vi "Icon Merge Layers.vi"(8 "error in (no error)":errorcluster, 11 "VI Refnum in":refnum<vi>) -> (0 "error out":errorcluster, 3 "VI Refnum out":refnum<vi>)   [LabVIEW 2019, in "Builtins.lvlib"]
doc: "Merges all VI icon layers to avoid icon template collisions.\n\nCreated by: Ryan Pacini"
uses:
  Builtins.lvlib
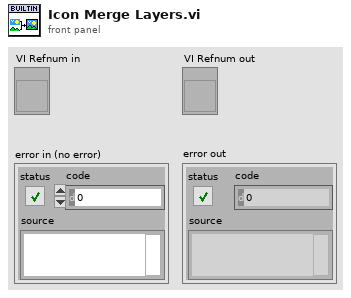
[diagram p1: front panel]
types:
  T1 = typedef "imagedata.ctl" = cluster{"image type":i32, "image depth":i32, "image":u8[], "mask":u8[], "colors":u32[], "Rectangle":cluster{"left":i16, "top":i16, "right":i16, "bottom":i16}}
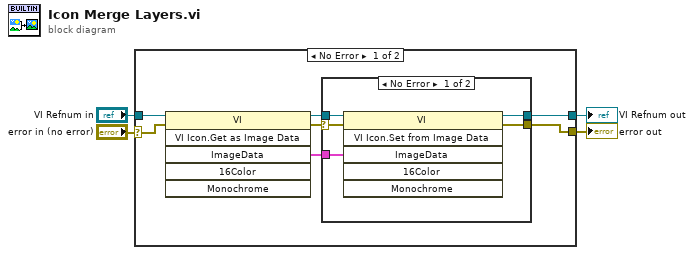
[diagram p0: block diagram]
diagram:
  n1 = case shown="No Error" "error in (no error)" {
    selector: "error in (no error)" -> [w11 w19]
    tunnel: "VI Refnum in" -> [w10 w20]
    tunnel: [w9 w20] -> w2
    tunnel: [w5 w19] -> w1
    frame No Error {
      n2 = invoke class="VI" method="VI Icon.Get as Image Data"(reference=w10, error in=w11) -> (reference out=w6:refnum<vi>, error out=w8:errorcluster, "ImageData"=w7:T1)  [unwired: 4 in, 3 out]
      n3 = case shown="No Error" w8 {
        selector: w8 -> [w14 w18]
        tunnel: w6 -> [w16 w17]
        tunnel: w7 -> [w15 _]
        tunnel: [w13 w18] -> w5
        tunnel: [w12 w17] -> w9
        frame No Error {
          n4 = invoke class="VI" method="VI Icon.Set from Image Data"(reference=w16, error in=w14, "ImageData"=w15) -> (reference out=w12:refnum<vi>, error out=w13:errorcluster)  [unwired: 3 in, 4 out]
        }
        frame Error {
        }
      }
    }
    frame Error {
    }
  }
  "VI Refnum out" <- w2
  "error out" <- w1
